vi "俄罗斯方块.vi"() -> ()   [LabVIEW 2016]
uses:
  <vilib>/Utility/config.llb/Read Key (String).vi
  <vilib>/Utility/config.llb/Write Key (String).vi
  <vilib>/Utility/config.llb/NI_LVConfig.lvlib
panel:
  out "配置文件路径":path
  out "结束状态":bool=TRUE
  out "落下状态":bool=TRUE
  in  "下落触发源":bool=TRUE
  out "速度":i32
  in  "开始/暂停":bool
  out "最多行数":string
  out "最高分数":string
  out "行数":string
  out "分数":string
  in  "退出":bool
  out "当前形状数组":u32[][](array[colorbox])
  out "Y":i8
  out "X":i8
  out "颜色盒":u32(colorbox)
  in  "新形状触发源":bool=TRUE
  in  "绘图触发源":bool=TRUE
  out "新形状数组":u32[][](array[colorbox])
  out "主窗数组":u32[][](array[colorbox])
  out "二维图片":picture
  # "上方向键：变形\n左方向键：左移\n右方向键：右移\n下方向键：下移\n空　　格：落下"
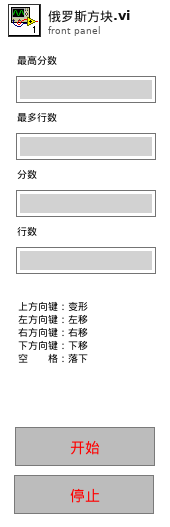
[diagram p1: front panel]
types:
  T1 = typedef "NI_LVConfig.lvlib/Config Data RefNum.ctl" = refnum<k1>
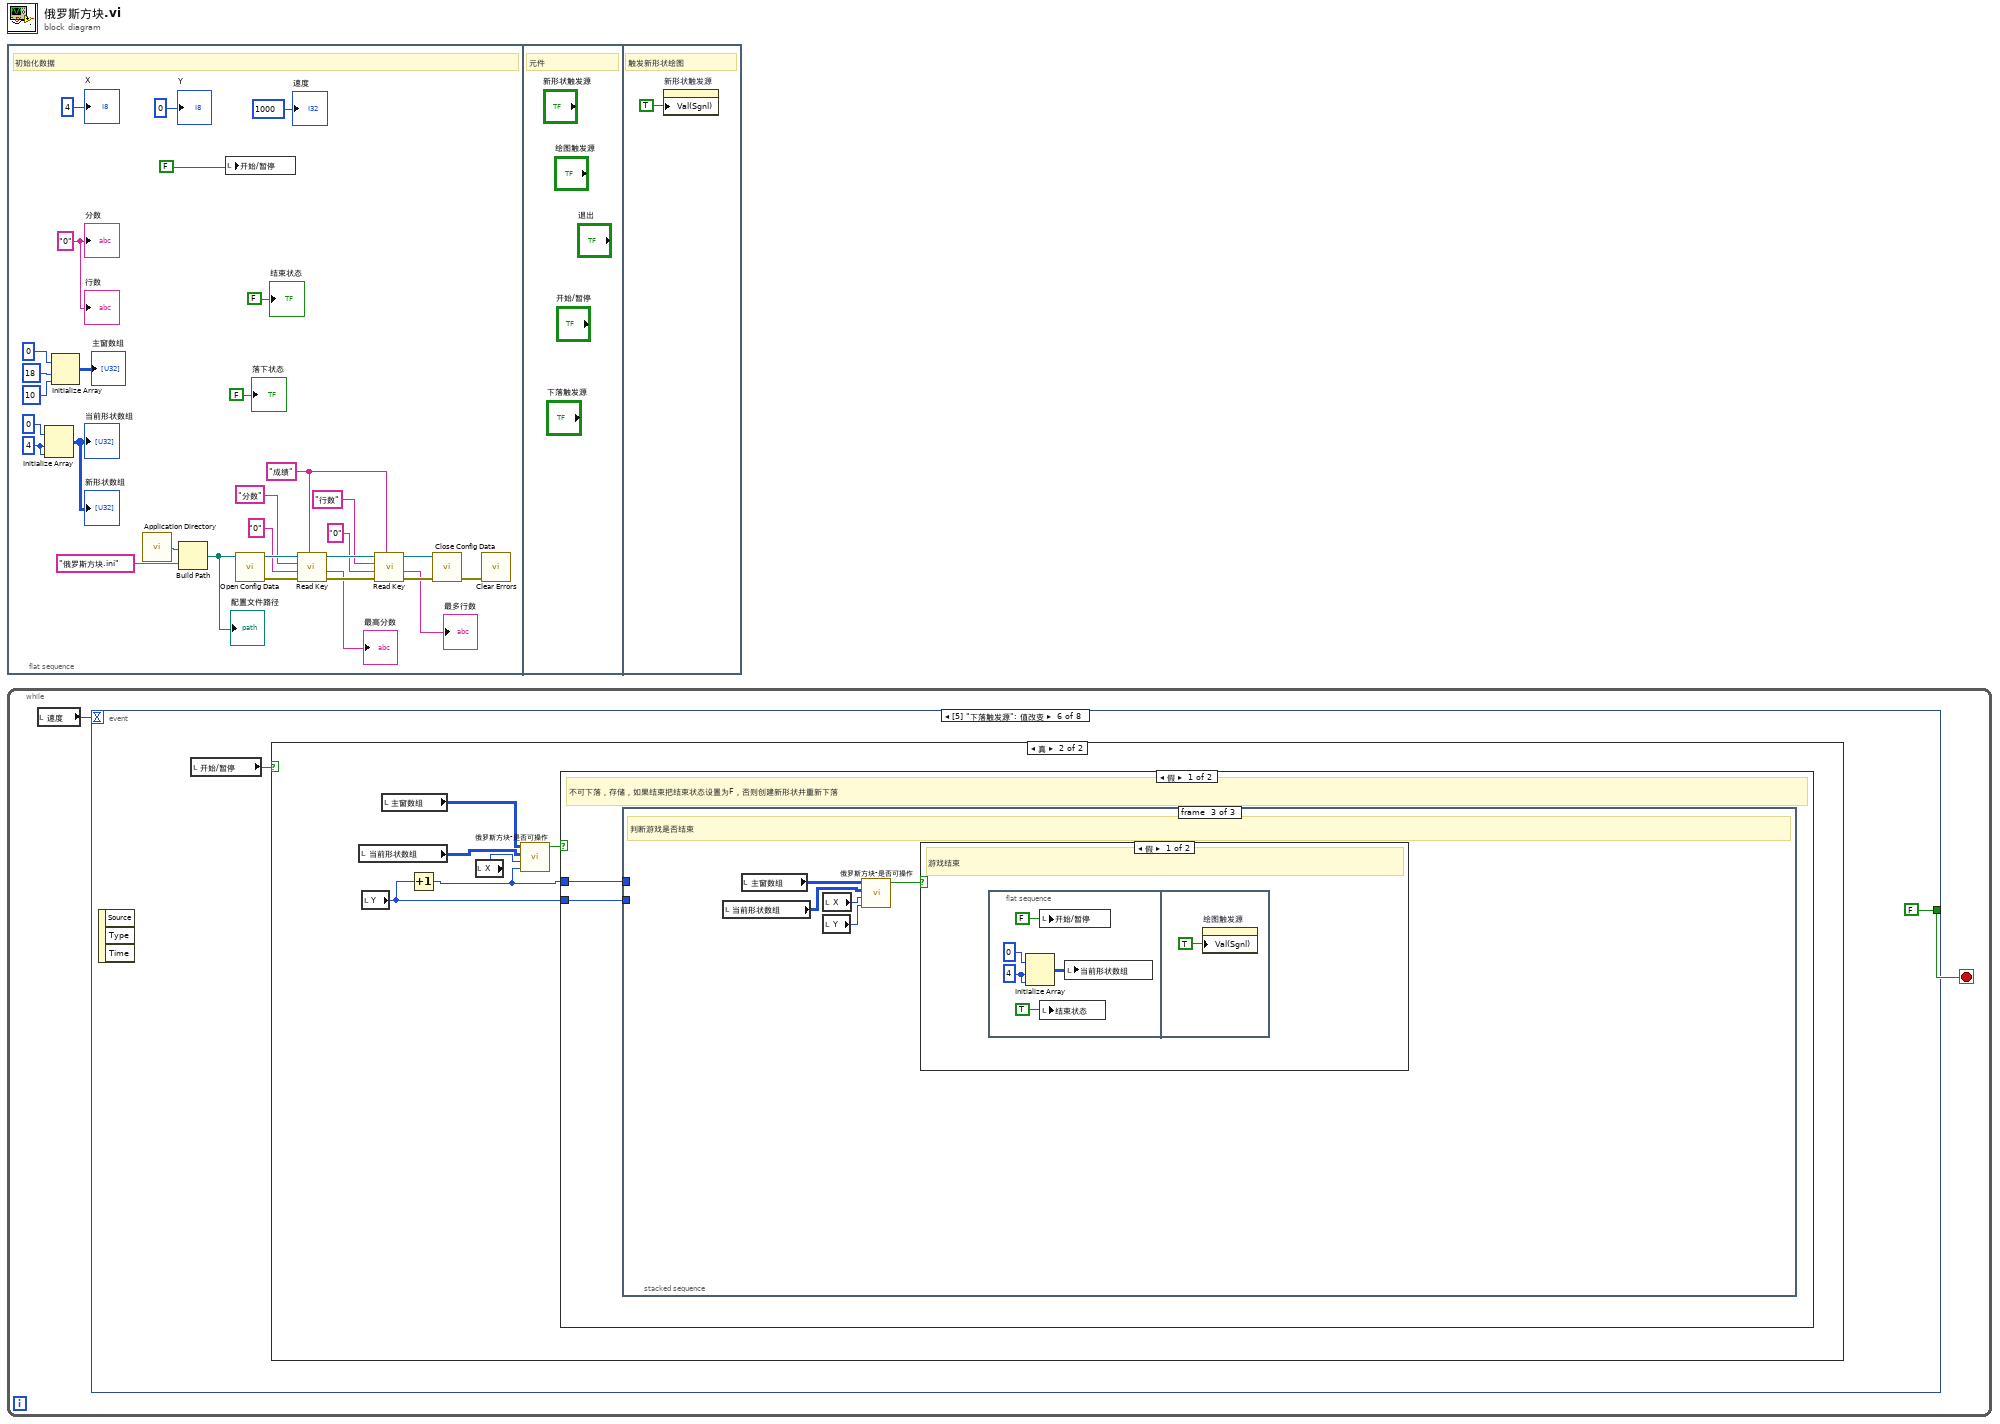
[diagram p0: block diagram]
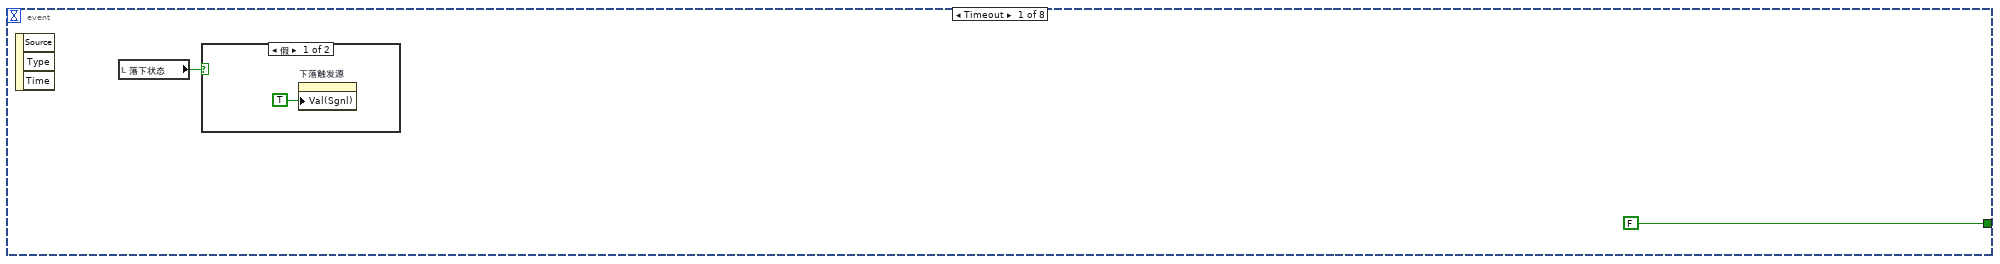
[diagram p2: hidden frame]
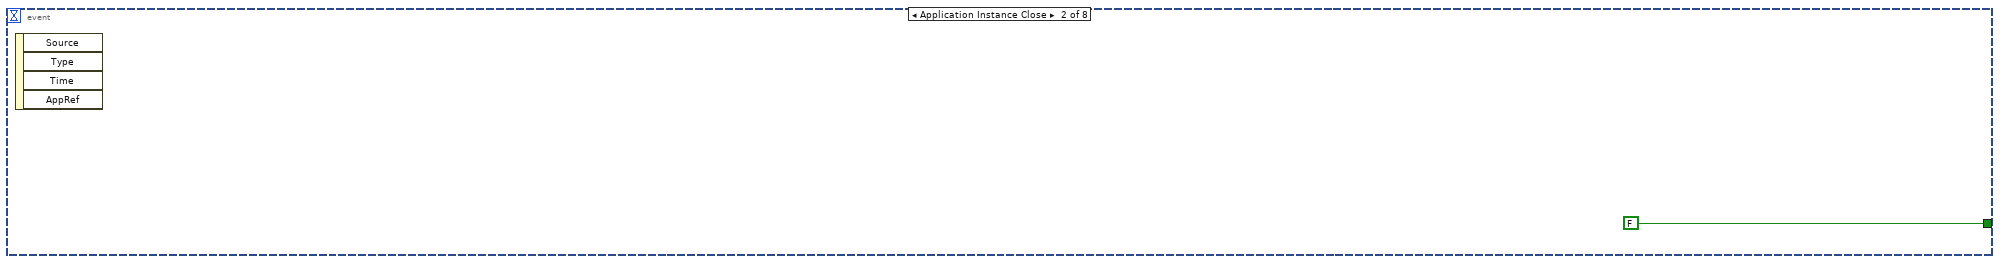
[diagram p4: hidden frame]
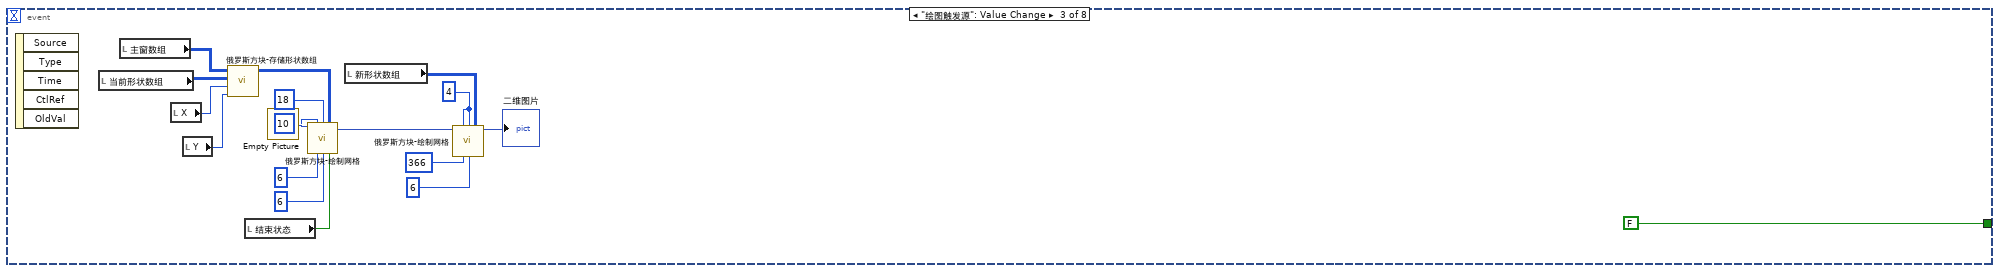
[diagram p5: hidden frame]
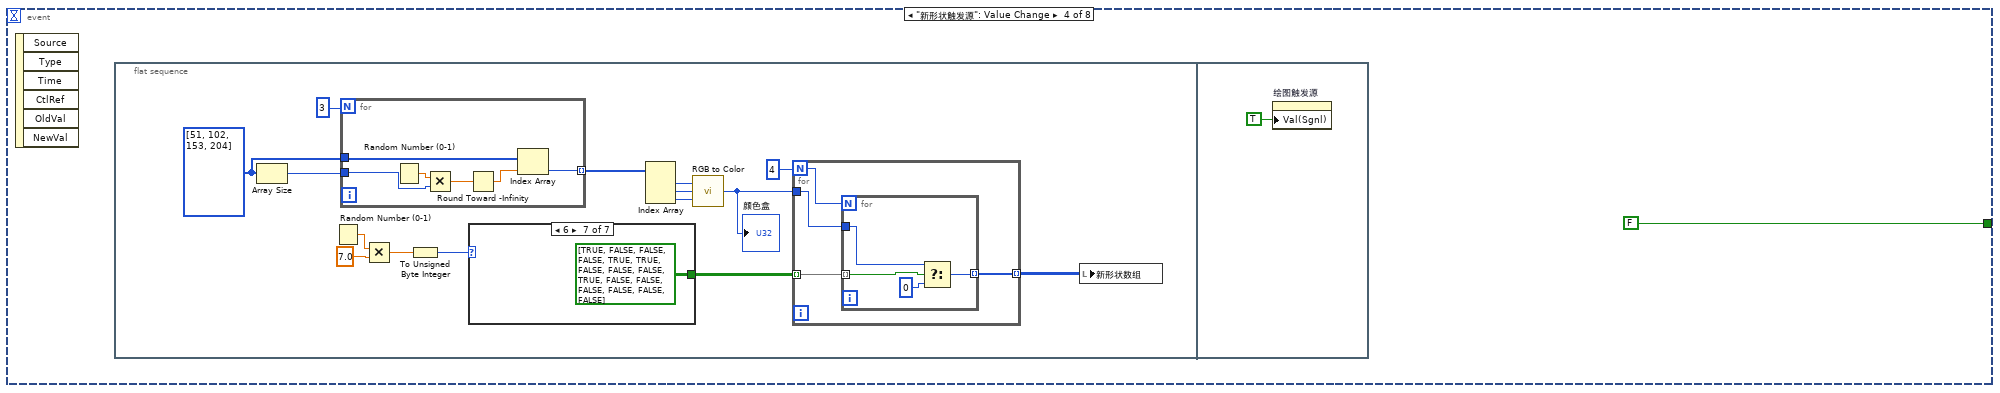
[diagram p6: hidden frame]
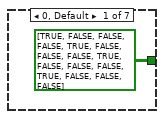
[diagram p7: hidden frame]
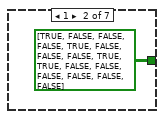
[diagram p8: hidden frame]
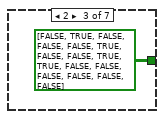
[diagram p9: hidden frame]
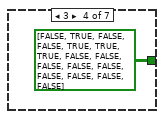
[diagram p10: hidden frame]
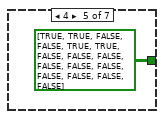
[diagram p11: hidden frame]
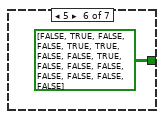
[diagram p12: hidden frame]
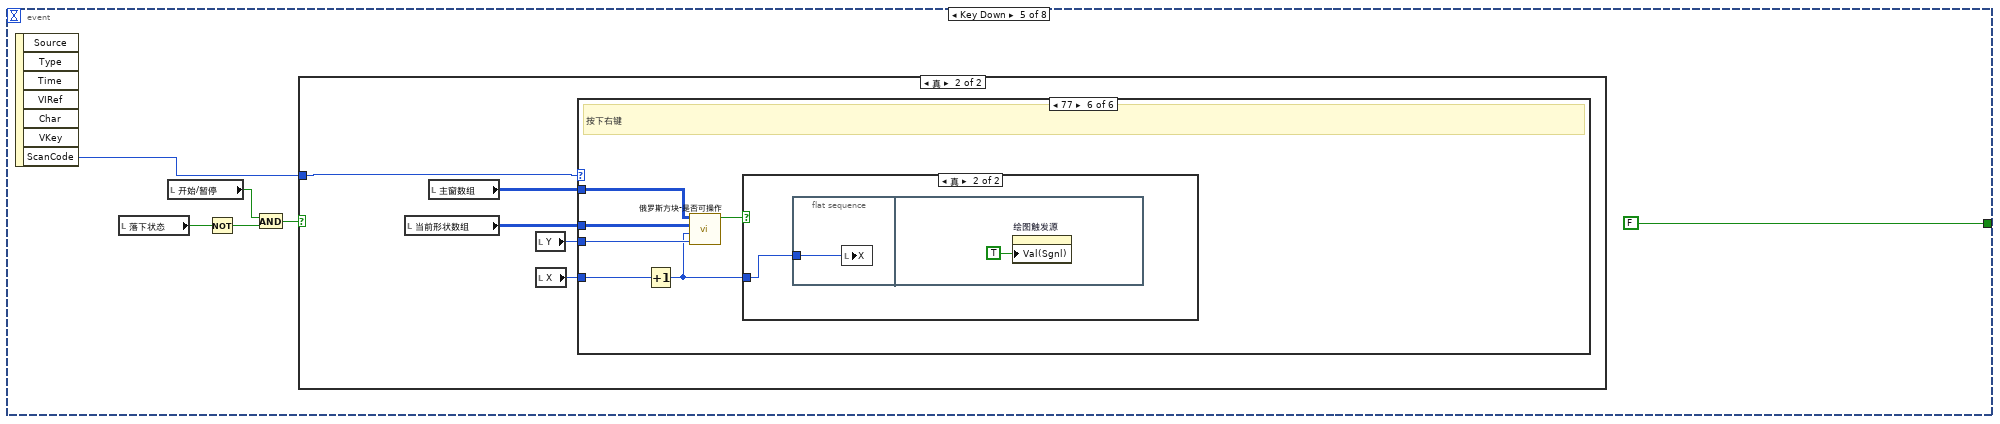
[diagram p13: hidden frame]
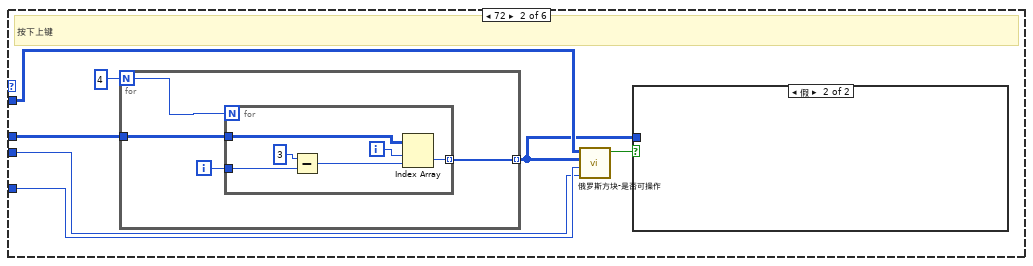
[diagram p16: hidden frame]
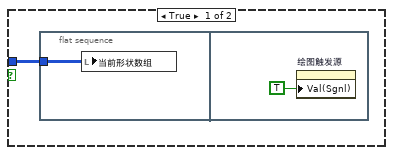
[diagram p17: hidden frame]
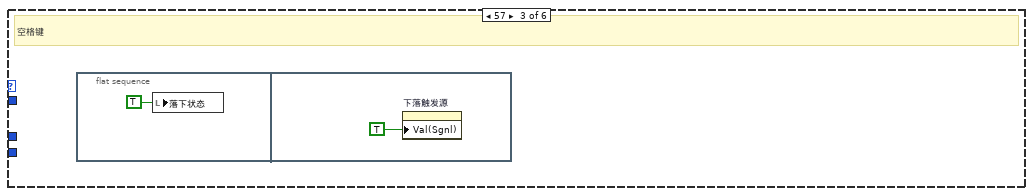
[diagram p18: hidden frame]
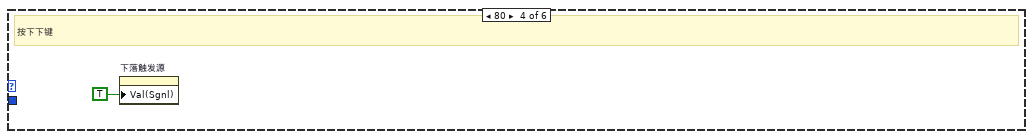
[diagram p19: hidden frame]
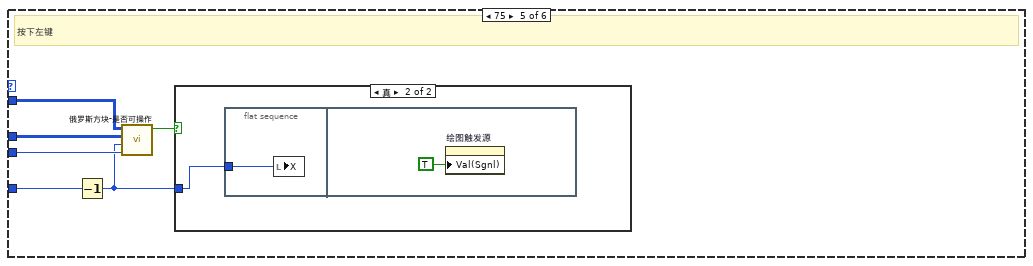
[diagram p20: hidden frame]
diagram:
  n1 = flat-sequence {
    frame #0 {
      w6 = "成绩" ("section")
      w22 = "0" ("行数")
      w24 = 4 ("维数大小")
      # "初始化数据"
      n2 = Initialize Array(u32 0 ("元素"), w24, w24) -> (→"新形状数组" →"当前形状数组":u32[][])
      n3 = Initialize Array(u32 0 ("元素"), 18 ("维数大小"), 10 ("维数大小")) -> (→"主窗数组":u32[][])
      n4 = call <vilib>:"Application Directory.vi"() -> ("Application Directory"=w5:path)
      n5 = Build Path(base path=w5, name or relative path="俄罗斯方块.ini" ("名称或相对路径")) -> (appended path=w10:path)
      "配置文件路径" <- w10
      n6 = local write "开始/暂停"(FALSE ("运行状态")) -> ()
      n7 = call <vilib>:"Open Config Data.vi"("configuration file path"=w10) -> ("error out"=w12:errorcluster, "refnum"=w21:T1)  [unwired: 8 in, 1 out]
      n8 = call-poly <vilib>:"Read Key.vi"("section"=w6, "error in (no error)"=w12, "default value"="0", "key"="分数", "refnum"=w21) -> ("error out"=w13:errorcluster, "value"=→"最高分数":string, "refnum out"=w18:T1)  [unwired: 3 in, 1 out]
      n9 = call-poly <vilib>:"Read Key.vi"("section"=w6, "error in (no error)"=w13, "default value"="0", "key"="行数", "refnum"=w18) -> ("error out"=w14:errorcluster, "value"=→"最多行数":string, "refnum out"=w15:T1)  [unwired: 3 in, 1 out]
      n10 = call <vilib>:"Close Config Data.vi"("error in (no error)"=w14, "refnum"=w15) -> ("error out"=w7:errorcluster)  [unwired: 8 in, 1 out]
      n11 = call <vilib>:"Clear Errors.vi"("error in (no error)"=w7) -> ()  [unwired: 5 in, 2 out]
      "X" <- i8 4 ("X")
      "Y" <- i8 0 ("Y")
      "分数" <- w22
      "行数" <- w22
      "速度" <- 1000 ("速度")
      "落下状态" <- FALSE ("落下状态")
      "结束状态" <- FALSE ("结束状态")
    }
    frame #1 {
      # "元件"
    }
    frame #2 {
      # "触发新形状绘图"
      n12 = property on="新形状触发源" class="Bool (严格)"("Val(Sgnl)"=TRUE ("值(信号)")) -> ()  [unwired: 2 in, 2 out]
    }
  }
  n13 = while {
    stop <- w34 stop-if-true
    n14 = local read "速度"() -> (w33:i32)
    n15 = event shown="[5] \"下落触发源\": 值改变" {
      selector: _ -> [_ _ _ _ _ _ _ _]
      dyn-events: _ -> [_ _ _ _ _ _ _ _]
      timeout: w33 -> [_ _ _ _ _ _ _ _]
      tunnel: [FALSE FALSE FALSE FALSE FALSE FALSE _ TRUE] -> w34
      event Timeout {
        n16 = event-data() -> ()  [unwired: 1 in, 3 out]
        n17 = local read "落下状态"() -> (w35:bool)
        n18 = case shown="假" w35 {
          frame False {
            n19 = property on="下落触发源" class="Bool (严格)"("Val(Sgnl)"=TRUE ("值(信号)")) -> ()  [unwired: 2 in, 2 out]
          }
          frame True {
          }
        }
      }
      event Application Instance Close {
        n20 = event-data() -> ()  [unwired: 1 in, 4 out]
      }
      event "绘图触发源": Value Change {
        w42 = i16 4 ("yN")
        n21 = event-data() -> ()  [unwired: 1 in, 5 out]
        n22 = local read "当前形状数组"() -> (w49:u32[][])
        n23 = local read "主窗数组"() -> (w46:u32[][])
        n24 = local read "X"() -> (w48:i8)
        n25 = local read "Y"() -> (w47:i8)
        n26 = call "俄罗斯方块-存储形状数组.vi"("Y"=w47, "X"=w48, "当前形状数组"=w49, "主窗数组输入"=w46) -> ("主窗数组输出"=w43:u32[][])  [unwired: 5 in]
        n27 = local read "结束状态"() -> (w39:bool)
        n28 = call "Empty Picture"() -> ("empty picture"=w53:picture)
        n29 = call "俄罗斯方块-绘制网格.vi"("图片输入"=w53, "xN"=i16 10, "yN"=i16 18, "数组"=w43, "xOffset"=i16 6, "yOffset"=i16 6, "结束状态"=w39) -> ("图片输出"=w55:picture)  [unwired: 8 in]
        n30 = local read "新形状数组"() -> (w41:u32[][])
        n31 = call "俄罗斯方块-绘制网格.vi"("图片输入"=w55, "xN"=w42, "yN"=w42, "数组"=w41, "xOffset"=i16 366, "yOffset"=i16 6) -> ("图片输出"=→"二维图片":picture)  [unwired: 9 in]
      }
      event "新形状触发源": Value Change {
        n32 = event-data() -> ()  [unwired: 1 in, 6 out]
        n33 = flat-sequence {
          frame #0 {
            w60 = u8[] [51, 102, 153, 204]
            n34 = Array Size(array=w60) -> (size(s)=w61:i32)
            n35 = Random Number (0-1)() -> (number: 0 to 1=w66:dbl)
            n36 = for {
              N: 3 -> [_]
              tunnel: [w90] -> w71 mode=indexing
              tunnel: w61 -> [w92]
              tunnel: w60 -> [w91]
              n37 = Random Number (0-1)() -> (number: 0 to 1=w93:dbl)
              n38 = Multiply(x=w93, y=w92) -> (x*y=w88:dbl)
              n39 = Round Toward -Infinity(1:w88) -> (0:w89:dbl)
              n40 = Index Array(array=w91, index=w89) -> (element=w90:u8)
            }
            n41 = Multiply(x=w66, y=7.0) -> (x*y=w65:dbl)
            n42 = To Unsigned Byte Integer(number=w65) -> (unsigned 8bit integer=w67:u8)
            n43 = case shown="6" w67 {
              tunnel: [bool[][] [[TRUE, FALSE, FALSE, FALSE], [TRUE, FALSE, FALSE, FALSE], [TRUE, FALSE, FALSE, FALSE], [TRUE, FALSE, FALSE, FALSE]] bool[][] [[TRUE, FALSE, FALSE, FALSE], [TRUE, FALSE, FALSE, FALSE], [TRUE, TRUE, FALSE, FALSE], [FALSE, FALSE, FALSE, FALSE]] bool[][] [[FALSE, TRUE, FALSE, FALSE], [FALSE, TRUE, FALSE, FALSE], [TRUE, TRUE, FALSE, FALSE], [FALSE, FALSE, FALSE, FALSE]] bool[][] [[FALSE, TRUE, FALSE, FALSE], [TRUE, TRUE, TRUE, FALSE], [FALSE, FALSE, FALSE, FALSE], [FALSE, FALSE, FALSE, FALSE]] bool[][] [[TRUE, TRUE, FALSE, FALSE], [TRUE, TRUE, FALSE, FALSE], [FALSE, FALSE, FALSE, FALSE], [FALSE, FALSE, FALSE, FALSE]] bool[][] [[FALSE, TRUE, FALSE, FALSE], [TRUE, TRUE, FALSE, FALSE], [TRUE, FALSE, FALSE, FALSE], [FALSE, FALSE, FALSE, FALSE]] bool[][] [[TRUE, FALSE, FALSE, FALSE], [TRUE, TRUE, FALSE, FALSE], [FALSE, TRUE, FALSE, FALSE], [FALSE, FALSE, FALSE, FALSE]]] -> w62
              frame 0, Default {
              }
              frame 1 {
              }
              frame 2 {
              }
              frame 3 {
              }
              frame 4 {
              }
              frame 5 {
              }
              frame 6 {
              }
            }
            n44 = Index Array(array=w71) -> (element #1=w70:u8, element #2=w69:u8, element #3=w68:u8)  [unwired: 3 in]
            n45 = call <vilib>:"RGB to Color.vi"("B"=w68, "G"=w69, "R"=w70) -> ("Color"=w59:u32)
            "颜色盒" <- w59
            n46 = for {
              N: 4 -> [w73]
              tunnel: w59 -> [w76]
              tunnel: w62 -> [w75] mode=indexing
              tunnel: [w74] -> w58 mode=indexing
              n47 = for {
                N: w73 -> [_]
                tunnel: w76 -> [w80]
                tunnel: w75 -> [w78] mode=indexing
                tunnel: [w77] -> w74 mode=indexing
                n48 = Select(t=w80, s=w78, f=u32 0) -> (s? t:f=w77:u32)
              }
            }
            n49 = local write "新形状数组"(w58) -> ()
          }
          frame #1 {
            n50 = property on="绘图触发源" class="Bool (严格)"("Val(Sgnl)"=TRUE ("绘图触发源")) -> ()  [unwired: 2 in, 2 out]
          }
        }
      }
      event Key Down {
        n51 = event-data() -> ("ScanCode"=w99:i16)  [unwired: 1 in, 6 out]
        n52 = local read "落下状态"() -> (w95:bool)
        n53 = local read "开始/暂停"() -> (w97:bool)
        n54 = Not(x=w95) -> (.not. x?=w96:bool)
        n55 = And(x=w97, y=w96) -> (x .and. y?=w98:bool)
        n56 = case shown="真" w98 {
          tunnel: w99 -> [_ w105]
          frame False {
          }
          frame True {
            n57 = local read "当前形状数组"() -> (w103:u32[][])
            n58 = local read "主窗数组"() -> (w104:u32[][])
            n59 = local read "Y"() -> (w101:i8)
            n60 = local read "X"() -> (w102:i8)
            n61 = case shown="77" w105 {
              tunnel: w104 -> [_ w112 _ _ w133 w142]
              tunnel: w103 -> [_ w107 _ _ w132 w141]
              tunnel: w102 -> [_ w111 _ _ w130 w139]
              tunnel: w101 -> [_ w110 _ _ w131 w140]
              frame 0, Default {
              }
              frame 72 {
                # "按下上键"
                n62 = for {
                  N: 4 -> [w115]
                  tunnel: [w116] -> w106 mode=indexing
                  tunnel: w107 -> [w114]
                  i -> [w113]
                  n63 = for {
                    N: w115 -> [_]
                    tunnel: [w122] -> w116 mode=indexing
                    tunnel: w114 -> [w121]
                    tunnel: w113 -> [w117]
                    i -> [w118]
                    n64 = Subtract(x=i8 3, y=w117) -> (x-y=w119:i32)
                    n65 = Index Array(array=w121, index (row)=w118, index (col)=w119) -> (element=w122:u32)
                  }
                }
                n66 = call "俄罗斯方块-是否可操作.vi"("Y"=w110, "X"=w111, "形状数组"=w106, "主窗数组"=w112) -> ("是否可操作"=w109:bool)  [unwired: 7 in]
                n67 = case shown="假" w109 {
                  tunnel: w106 -> [w123 _]
                  frame True {
                    n68 = flat-sequence {
                      tunnel: w123 -> [w124]
                      frame #0 {
                        n69 = local write "当前形状数组"(w124) -> ()
                      }
                      frame #1 {
                        n70 = property on="绘图触发源" class="Bool (严格)"("Val(Sgnl)"=TRUE ("值(信号)")) -> ()  [unwired: 2 in, 2 out]
                      }
                    }
                  }
                  frame False {
                  }
                }
              }
              frame 57 {
                # "空格键"
                n71 = flat-sequence {
                  frame #0 {
                    n72 = local write "落下状态"(TRUE ("落下状态")) -> ()
                  }
                  frame #1 {
                    n73 = property on="下落触发源" class="Bool (严格)"("Val(Sgnl)"=TRUE ("值(信号)")) -> ()  [unwired: 2 in, 2 out]
                  }
                }
              }
              frame 80 {
                # "按下下键"
                n74 = property on="下落触发源" class="Bool (严格)"("Val(Sgnl)"=TRUE ("值(信号)")) -> ()  [unwired: 2 in, 2 out]
              }
              frame 75 {
                # "按下左键"
                n75 = Decrement(x=w130) -> (x-1=w129:i8)
                n76 = call "俄罗斯方块-是否可操作.vi"("Y"=w131, "X"=w129, "形状数组"=w132, "主窗数组"=w133) -> ("是否可操作"=w134:bool)  [unwired: 7 in]
                n77 = case shown="真" w134 {
                  tunnel: w129 -> [_ w135]
                  frame False {
                  }
                  frame True {
                    n78 = flat-sequence {
                      tunnel: w135 -> [w136]
                      frame #0 {
                        n79 = local write "X"(w136) -> ()
                      }
                      frame #1 {
                        n80 = property on="绘图触发源" class="Bool (严格)"("Val(Sgnl)"=TRUE ("值(信号)")) -> ()  [unwired: 2 in, 2 out]
                      }
                    }
                  }
                }
              }
              frame 77 {
                # "按下右键"
                n81 = Increment(x=w139) -> (x+1=w138:i8)
                n82 = call "俄罗斯方块-是否可操作.vi"("Y"=w140, "X"=w138, "形状数组"=w141, "主窗数组"=w142) -> ("是否可操作"=w143:bool)  [unwired: 7 in]
                n83 = case shown="真" w143 {
                  tunnel: w138 -> [_ w144]
                  frame False {
                  }
                  frame True {
                    n84 = flat-sequence {
                      tunnel: w144 -> [w145]
                      frame #0 {
                        n85 = local write "X"(w145) -> ()
                      }
                      frame #1 {
                        n86 = property on="绘图触发源" class="Bool (严格)"("Val(Sgnl)"=TRUE ("值(信号)")) -> ()  [unwired: 2 in, 2 out]
                      }
                    }
                  }
                }
              }
            }
          }
        }
      }
      event "下落触发源": Value Change {
        n87 = event-data() -> ()  [unwired: 1 in, 3 out]
        n88 = local read "开始/暂停"() -> (w147:bool)
        n89 = case shown="真" w147 {
          frame False {
          }
          frame True {
            n90 = local read "当前形状数组"() -> (w153:u32[][])
            n91 = local read "Y"() -> (w151:i8)
            n92 = local read "主窗数组"() -> (w154:u32[][])
            n93 = Increment(x=w151) -> (x+1=w149:i8)
            n94 = local read "X"() -> (w152:i8)
            n95 = call "俄罗斯方块-是否可操作.vi"("Y"=w149, "X"=w152, "形状数组"=w153, "主窗数组"=w154) -> ("是否可操作"=w150:bool)  [unwired: 7 in]
            n96 = case shown="假" w150 {
              tunnel: w149 -> [w156 w220]
              tunnel: w151 -> [w155 _]
              frame False {
                # "不可下落，存储，如果结束把结束状态设置为F，否则创建新形状并重新下落"
                n97 = stacked-sequence {
                  tunnel: w156 -> [_ _ _]
                  tunnel: w155 -> [w162 _ _]
                  frame #0 {
                    # "存储并消除满行和记分"
                    n98 = local read "当前形状数组"() -> (w165:u32[][])
                    n99 = local read "主窗数组"() -> (w164:u32[][])
                    n100 = local read "X"() -> (w163:i8)
                    n101 = call "俄罗斯方块-存储形状数组.vi"("Y"=w162, "X"=w163, "当前形状数组"=w165, "主窗数组输入"=w164) -> ("主窗数组输出"=w161:u32[][])  [unwired: 5 in]
                    n102 = call "俄罗斯方块-消除满行.vi"("输入数组"=w161) -> ("行数"=w157:u32, "分数"=w158:u32, "输出数组"=w160:u32[][])  [unwired: 8 in]
                    n103 = Greater Than 0?(x=w157) -> (x > 0?=w159:bool)
                    n104 = local write "主窗数组"(w160) -> ()
                    n105 = case shown="真" w159 {
                      tunnel: w158 -> [_ w181]
                      tunnel: w157 -> [_ w182]
                      frame False {
                      }
                      frame True {
                        n106 = local read "分数"() -> (w180:string)
                        n107 = local read "行数"() -> (w177:string)
                        n108 = local read "最多行数"() -> (w173:string)
                        n109 = local read "最高分数"() -> (w174:string)
                        n110 = Decimal String To Number(string=w180) -> (number=w176:i32)  [unwired: 2 in, 1 out]
                        n111 = Decimal String To Number(string=w177) -> (number=w175:i32)  [unwired: 2 in, 1 out]
                        n112 = Decimal String To Number(string=w173) -> (number=w166:i32)  [unwired: 2 in, 1 out]
                        n113 = Decimal String To Number(string=w174) -> (number=w170:i32)  [unwired: 2 in, 1 out]
                        n114 = Add(x=w181, y=w176) -> (x+y=w169:u32)
                        n115 = Add(x=w175, y=w182) -> (x+y=w167:u32)
                        n116 = Greater?(x=w169, y=w170) -> (0:w171:bool)
                        n117 = Greater?(x=w167, y=w166) -> (0:w168:bool)
                        n118 = Number To Decimal String(number=w169) -> (decimal integer string=w179:string)  [unwired: 1 in]
                        n119 = Number To Decimal String(number=w167) -> (decimal integer string=w178:string)  [unwired: 1 in]
                        n120 = Or(x=w171, y=w168) -> (x .or. y?=w172:bool)
                        n121 = local write "分数"(w179) -> ()
                        n122 = local write "行数"(w178) -> ()
                        n123 = case shown="真" w172 {
                          tunnel: w171 -> [_ w202]
                          tunnel: w169 -> [_ w201]
                          tunnel: w170 -> [_ w200]
                          tunnel: w168 -> [_ w198]
                          tunnel: w167 -> [_ w197]
                          tunnel: w166 -> [_ w196]
                          frame False {
                          }
                          frame True {
                            w187 = "成绩" ("section")
                            n124 = Select(t=w201, s=w202, f=w200) -> (s? t:f=w203:u32)
                            n125 = Select(t=w197, s=w198, f=w196) -> (s? t:f=w199:u32)
                            n126 = local read "配置文件路径"() -> (w195:path)
                            n127 = Number To Decimal String(number=w199) -> (decimal integer string=w185:string)  [unwired: 1 in]
                            n128 = Number To Decimal String(number=w203) -> (decimal integer string=w183:string)  [unwired: 1 in]
                            n129 = local write "最高分数"(w183) -> ()
                            n130 = local write "最多行数"(w185) -> ()
                            n131 = call <vilib>:"Open Config Data.vi"("configuration file path"=w195) -> ("error out"=w188:errorcluster, "refnum"=w189:T1)  [unwired: 8 in, 1 out]
                            n132 = call-poly <vilib>:"Write Key.vi"("section"=w187, "error in (no error)"=w188, "value"=w185, "key"="行数", "refnum"=w189) -> ("error out"=w190:errorcluster, "refnum out"=w191:T1)  [unwired: 4 in, 1 out]
                            n133 = call-poly <vilib>:"Write Key.vi"("section"=w187, "error in (no error)"=w190, "value"=w183, "key"="分数", "refnum"=w191) -> ("error out"=w192:errorcluster, "refnum out"=w193:T1)  [unwired: 4 in, 1 out]
                            n134 = call <vilib>:"Close Config Data.vi"("error in (no error)"=w192, "refnum"=w193) -> ("error out"=w194:errorcluster)  [unwired: 8 in, 1 out]
                            n135 = call <vilib>:"Clear Errors.vi"("error in (no error)"=w194) -> ()  [unwired: 5 in, 2 out]
                          }
                        }
                      }
                    }
                  }
                  frame #1 {
                    # "初始化落下状态、XY坐标、把新形状作为当前形状"
                    n136 = local read "新形状数组"() -> (w205:u32[][])
                    n137 = local write "落下状态"(FALSE ("落下状态")) -> ()
                    n138 = local write "当前形状数组"(w205) -> ()
                    n139 = local write "X"(i8 4 ("X")) -> ()
                    n140 = local write "Y"(i8 0 ("Y")) -> ()
                  }
                  frame #2 {
                    # "判断游戏是否结束"
                    n141 = local read "当前形状数组"() -> (w211:u32[][])
                    n142 = local read "主窗数组"() -> (w212:u32[][])
                    n143 = local read "X"() -> (w210:i8)
                    n144 = local read "Y"() -> (w209:i8)
                    n145 = call "俄罗斯方块-是否可操作.vi"("Y"=w209, "X"=w210, "形状数组"=w211, "主窗数组"=w212) -> ("是否可操作"=w208:bool)  [unwired: 7 in]
                    n146 = case shown="假" w208 {
                      frame False {
                        # "游戏结束"
                        n147 = flat-sequence {
                          frame #0 {
                            w216 = 4 ("维数大小")
                            n148 = Initialize Array(u32 0 ("元素"), w216, w216) -> (w214:u32[][])
                            n149 = local write "开始/暂停"(FALSE ("开始/暂停")) -> ()
                            n150 = local write "结束状态"(TRUE ("结束状态")) -> ()
                            n151 = local write "当前形状数组"(w214) -> ()
                          }
                          frame #1 {
                            n152 = property on="绘图触发源" class="Bool (严格)"("Val(Sgnl)"=TRUE ("值(信号)")) -> ()  [unwired: 2 in, 2 out]
                          }
                        }
                      }
                      frame True {
                        # "未结束，产生新形状数据"
                        n153 = property on="新形状触发源" class="Bool (严格)"("Val(Sgnl)"=TRUE ("值(信号)")) -> ()  [unwired: 2 in, 2 out]
                      }
                    }
                  }
                }
              }
              frame True {
                n154 = flat-sequence {
                  tunnel: w220 -> [w221]
                  frame #0 {
                    n155 = local write "Y"(w221) -> ()
                  }
                  frame #1 {
                    n156 = local read "落下状态"() -> (w222:bool)
                    n157 = case shown="假" w222 {
                      frame False {
                        n158 = property on="绘图触发源" class="Bool (严格)"("Val(Sgnl)"=FALSE ("值(信号)")) -> ()  [unwired: 2 in, 2 out]
                      }
                      frame True {
                        n159 = property on="下落触发源" class="Bool (严格)"("Val(Sgnl)"=TRUE ("值(信号)")) -> ()  [unwired: 2 in, 2 out]
                      }
                    }
                  }
                }
              }
            }
          }
        }
      }
      event "开始/暂停": Value Change {
        n160 = event-data() -> ()  [unwired: 1 in, 6 out]
        n161 = flat-sequence {
          frame #0 {
            n162 = local read "结束状态"() -> (w225:bool)
            n163 = local read "新形状数组"() -> (w226:u32[][])
            n164 = case shown="真" w225 {
              frame False {
              }
              frame True {
                n165 = Initialize Array(u32 0 ("元素"), 18 ("维数大小"), 10 ("维数大小")) -> (w227:u32[][])
                n166 = local write "主窗数组"(w227) -> ()
              }
            }
            n167 = local write "当前形状数组"(w226) -> ()
          }
          frame #1 {
            n168 = property on="新形状触发源" class="Bool (严格)"("Val(Sgnl)"=TRUE ("值(信号)")) -> ()  [unwired: 2 in, 2 out]
          }
        }
      }
      event "退出": Value Change {
        n169 = event-data() -> ()  [unwired: 1 in, 6 out]
      }
    }
  }
